vi "Dashboard Main.vi"() -> ()   [LabVIEW 2014]
uses:
  <vilib>/event_ctls.llb/eventvkey.ctl
  <vilib>/Rock Robotics/WPI/Dashboard/WPI_DashboardLogging Global.vi
  <vilib>/Rock Robotics/Network Tables/SD Read Number.vi
  <vilib>/Rock Robotics/Network Tables/SD Read Boolean Array.vi
  <vilib>/Rock Robotics/Network Tables/SD Read Boolean.vi
  <vilib>/Rock Robotics/Network Tables/SD Write Number.vi
  <vilib>/Rock Robotics/Network Tables/SD Write Boolean.vi
  <vilib>/Utility/config.llb/Write Key (String).vi
  <vilib>/Utility/config.llb/Write Key (I32).vi
  <vilib>/Utility/config.llb/NI_LVConfig.lvlib
panel:
  out "Gripper Open":bool
  out "Compresser Running":bool
  out "Camera 1":bool
  in  "TCP":refnum<k5>
  in  "Rec Mode":enum32{"Stop", "Record", "Playback"}(radio)
  in  "Vision":u16(ring)=2 items=["Camera Off", "USB Camera SW", "USB Camera HW", "IP Camera"]
  out "Camera IP":string
  out "Image Message":string="Timeout in Camera Communications"
  in  "Dashboard Tab":T1(tab)=enum."Drive"
  out "Inrange 2":bool
  out "Inrange 1":bool
  in  "Winch 2 Encoder reset":bool
  out "Lower Micro SW 2":bool
  out "Upper Micro SW 2":bool
  out "Manual Over-Rided Winch 2":bool=TRUE
  out "lower limit 2":dbl
  out "upper limit 2":dbl
  out "PV: 2":dbl(slide) scale=0.0..100.0
  in  "Winch 1 Encoder reset":bool
  out "Lower Micro SW":bool
  out "Upper Micro SW":bool
  out "Manual Over-Rided Winch 1":bool
  out "lower limit":dbl
  out "upper limit":dbl
  out "PV:":dbl(slide) scale=0.0..70.0
  out "SP:":dbl(slide) min=0.0 max=0.0 scale=0.0..75.0
  in  "Match Time":dbl=135.0
  out "Match Count Down":dbl=135.0 format="%#_4g"
  out "PICK UP":bool=TRUE
  out "Distance to Target":dbl(slide) scale=0.0..100.0
  in  "Autonomous Mode to run :":T2(ring)
  in  "Camera Settings":T3={"Frame Rate"=25, "Compression"=20, "Size"=0} {"Frame Rate" scale=1.0..30.0; "Size" items=["640x480", "320x240", "160x120"]}
  out "MotorChart R":cluster{"Numeric":dbl, "Numeric":dbl}(graph)
  out "MotorChart L":T4(graph)={"Numeric"=0.0, "Numeric"=0.0, "Battery V"=11.890625}
  out "MotorSliders R":cluster{"MotorSlide1":dbl, "MotorSlide2":dbl} {"MotorSlide2" scale=-1.0..1.0 scale format="%#_2e"; "MotorSlide1" scale=-1.0..1.0 scale format="%#_2e"}
  out "MotorSliders L":T5={"MotorSlide1"=0.0, "MotorSlide2"=0.0, "MotorSlide4 2"=11.890625} {"MotorSlide4 2" scale=0.0..14.0 scale format="%#_2e"; "MotorSlide2" scale=-1.0..1.0 scale format="%#_2e"; "MotorSlide1" scale=-1.0..1.0 scale format="%#_2e"}
  out "JS1 Z":dbl(slide) scale=-1.0..1.0 scale format="%#_2e"
  out "JS1 Graph":cluster{"X":dbl, "Y":dbl}[](graph)=[{"X"=0.047244094488188976, "Y"=-0.007874015748031496}]
  out "JS1 Buttons":T6
  out "JS2 Z":dbl(slide) scale=-1.0..1.0 scale format="%#_2e"
  out "JS2 Graph":cluster{"X":dbl, "Y":dbl}[](graph)=[{"X"=-0.015748031496062992, "Y"=-0.05511811023622047}]
  out "JS2 Buttons":T6
  out "Mode":T7(ring)
  in  "DB Camera Config":bool
  out "fps":dbl=13.440860215053762 format="%#.1g"
  out "Mbps":dbl=5.913673836823652 format="%#.1g"
  out "Mbps 2":bool
  out "Sonar Limit":dbl
  in  "DB/String 9":string
  in  "DB/String 8":string
  in  "DB/String 7":string
  in  "DB/String 6":string
  in  "DB/String 5":string
  in  "DB/String 4":string
  in  "DB/String 3":string
  in  "DB/String 2":string
  in  "DB/String 1":string
  in  "DB/String 0":string
  in  "DB/Slider 0":dbl(slide) scale=0.0..5.0
  in  "DB/Slider 1":dbl(slide) scale=0.0..5.0
  in  "DB/Slider 2":dbl(slide) scale=0.0..5.0
  in  "DB/Slider 3":dbl(slide) scale=0.0..5.0
  out "DB/LED 3":bool
  out "DB/LED 2":bool
  out "DB/LED 1":bool
  out "DB/LED 0":bool
  in  "DB/Button 3":bool
  in  "DB/Button 2":bool
  in  "DB/Button 1":bool
  in  "DB/Button 0":bool caption="New Name"
  in  "Test Slider":dbl(slide) scale=0.0..100.0 scale format="%#_3g"
  in  "On/Off":bool caption="Solenoid"
  in  "Test Name":u16(ring) items=["Select the test to run...", "Example Test", "-------------------------------", "List of tests is built in robot code.", "Replace with your own automated tests."]
  in  "Test Tree":string(tree)
  in  "Motor":cluster{"Value":dbl, "Enable":bool} {"Value" scale=-1.0..1.0 scale format="%#_3g"}
  out "Progress":T8 {"Test Progress" scale=0.0..100.0}
  in  "Rev/Fwd":cluster{"Forward":bool, "Reverse":bool}
  in  "Test Ring":u16(ring) items=["Monochrome", "Color"]
  in  "Listbox":i32(listbox)
  out "Tree":string(tree)
  out "Camera Image":T9(plugin-control)
  out "Boolean":bool=TRUE
  # "Left"
  # "Front"
  # "Right"
  # "Battery"
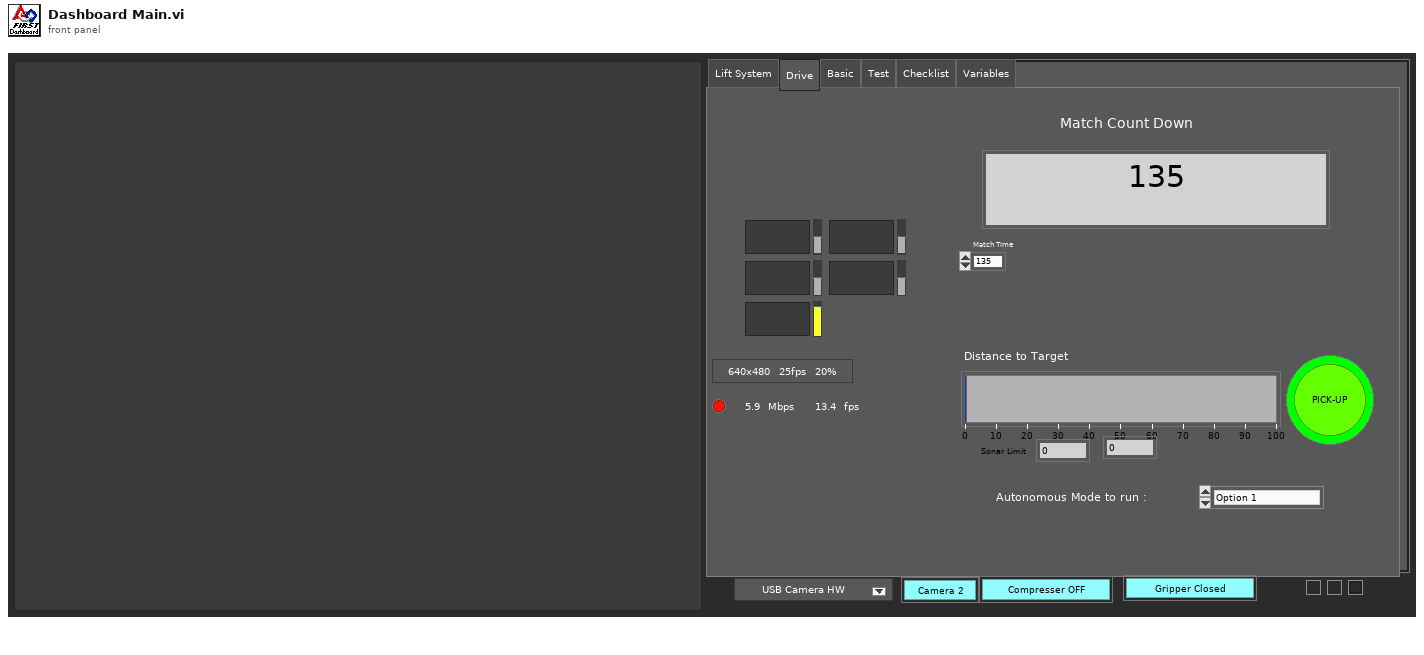
[diagram p1: front panel]
types:
  T1 = enum32{"Lift System", "Drive", "Basic", "Test", "Checklist", "Variables"}
  T2 = enum16{"Option 1", "Option 2", "Option 3", "Option 4", "Option 5", "Option 6"}
  T3 = cluster{"Frame Rate":i32, "Compression":i32, "Size":u16}
  T4 = cluster{"Numeric":dbl, "Numeric":dbl, "Battery V":dbl}
  T5 = cluster{"MotorSlide1":dbl, "MotorSlide2":dbl, "MotorSlide4 2":dbl}
  T6 = cluster{bool, bool, bool, bool, bool, bool, bool, bool, bool, bool, bool, bool}
  T7 = enum8{"Tele-Op Disabled", "Tele-Op Enabled", "Auto Disabled", "Auto Enabled", "Test Disabled", "Test Enabled", "Disconnected", "No Code", "E-Stop"}
  T8 = cluster{"Test Progress":u8, "Test Progress Text":string}
  T9 = typedef "IMAQ Image.ctl" = refnum<image>
  T10 = enum32{"Drive", "Basic", "Custom", "Test", "Checklist", "Variables"}
  T11 = typedef "Image Type" = u32
  T12 = cluster{"Camera Image":refnum<vi>, "Dashboard Tab":refnum<vi>, "Boolean":refnum<vi>, "Vision":refnum<vi>, "Rec Mode":refnum<vi>, "Test Slider":refnum<vi>, "On/Off ":refnum<vi>, "Test Ring":refnum<vi>, "Rev/Fwd":refnum<vi>, "Test Name":refnum<vi>, "Motor":refnum<vi>, "Progress":refnum<vi>, "CheckList":refnum<vi>, "Tree":refnum<vi>, "Test Tree":refnum<vi>}
  T13 = cluster{"Error Strings":string, "Disable Counts":cluster{u16, u16}, "Rail Faults":cluster{u16, u16, u16}, "Robot IP":string, "DB Mode":u8, "Event Info":cluster{"Name":string, "Type":u8, "Number":u16, "Replay":u8}, "Camera Addr":string}
  T14 = cluster{"Storage":cluster{"Disk Free":u64, "RAM Block":u32, "RAM free":u32}, "CPU Utilization":cluster{"CPU % ISR":sgl, "CPU % Time Crit":sgl, "CPU % Timed Str":sgl, "CPU % High":sgl, "CPU % Above":sgl, "CPU % Normal":sgl, "CPU % Low":sgl}, "CAN":cluster{"% Bus Utilization":sgl, "Bus Off Cnt":u32, "TX_FIFO Full Cnt":u32, "Receive Error Cnt":u8, "Transmit Error Cnt":u8}, "HID":cluster{"HID Outputs":u32, "Rumble Low":u16, "Rumble High":u16}[]}
  T15 = cluster{"Status bits":cluster{"Test Mode":bool, "Autonomous":bool, "Enabled":bool, "Code Start":bool, "Brownout":bool, "Reserved 2":bool, "Reserved 3":bool, "E-Stop":bool}, "Code Trace":cluster{"Disabled":bool, "TeleOp":bool, "Auto":bool, "Test":bool}, "Controller Type":enum16{"unknown", "cRIO", "roboRio"}, "Code?":enum16{"unknown", "noCode", "code"}, "Battery V":dbl}
  T16 = cluster{"Control Bits":cluster{"TestMode":bool, "Autonomous":bool, "Enabled":bool, "FMS Present":bool, bool, bool, bool, "E-Stop":bool}, "Team Station ":u8, "Countdown":sgl, "Joystick Values":cluster{"Axes":dbl[], "Buttons":bool[], "POVs":i16[]}[]}
  T17 = cluster{"Axes":dbl[], "Buttons":bool[], "POVs":i16[]}[]
  T18 = cluster{"Axes":dbl[], "Buttons":bool[], "POVs":i16[]}
  T19 = cluster{"Buttons[0]":bool, "Buttons[1]":bool, "Buttons[2]":bool, "Buttons[3]":bool, "Buttons[4]":bool, "Buttons[5]":bool, "Buttons[6]":bool, "Buttons[7]":bool, "Buttons[8]":bool, "Buttons[9]":bool, "Buttons[10]":bool, "Buttons[11]":bool}
  T20 = typedef "NI_LVConfig.lvlib/Config Data RefNum.ctl" = refnum<k1>
  T21 = cluster{"Operation":enum16{"Update", "Clear"}, "Color Box":u32}[]
  T22 = typedef "eventvkey.ctl" = enum16{"ASCII", "Enter", "Return", "Shift", "Ctrl", "Alt", "Cmd", "Opt", "Caps", "NumLock", "Clear", "Break", "Up", "Down", "Left", "Right", "Insert", "Delete", "Home", "End", "PageUp", "PageDown", "Escape", "Help", "Pause", "ScrollLock", "F1", "F2", "F3", "F4", "F5", "F6", "F7", "F8", "F9", "F10", "F11", "F12", "F13", "F14", "F15", "F16", "F17", "F18", "F19", "F20", "F21", "F22", "F23", "F24", "Play", "VolumeUp", "VolumeDown", "Mute", "Two Byte Char"}
  T23 = cluster{"Image Size":bool, "Image Type":bool, "Pixel Value":bool, "ROI Information":bool, "Zoom Factor":bool}
  T24 = enum8{"Enabled", "Disabled", "Disabled and Grayed Out"}
  T25 = cluster{"Operation":enum16{"Update", "Clear"}, "Color Box":u32}
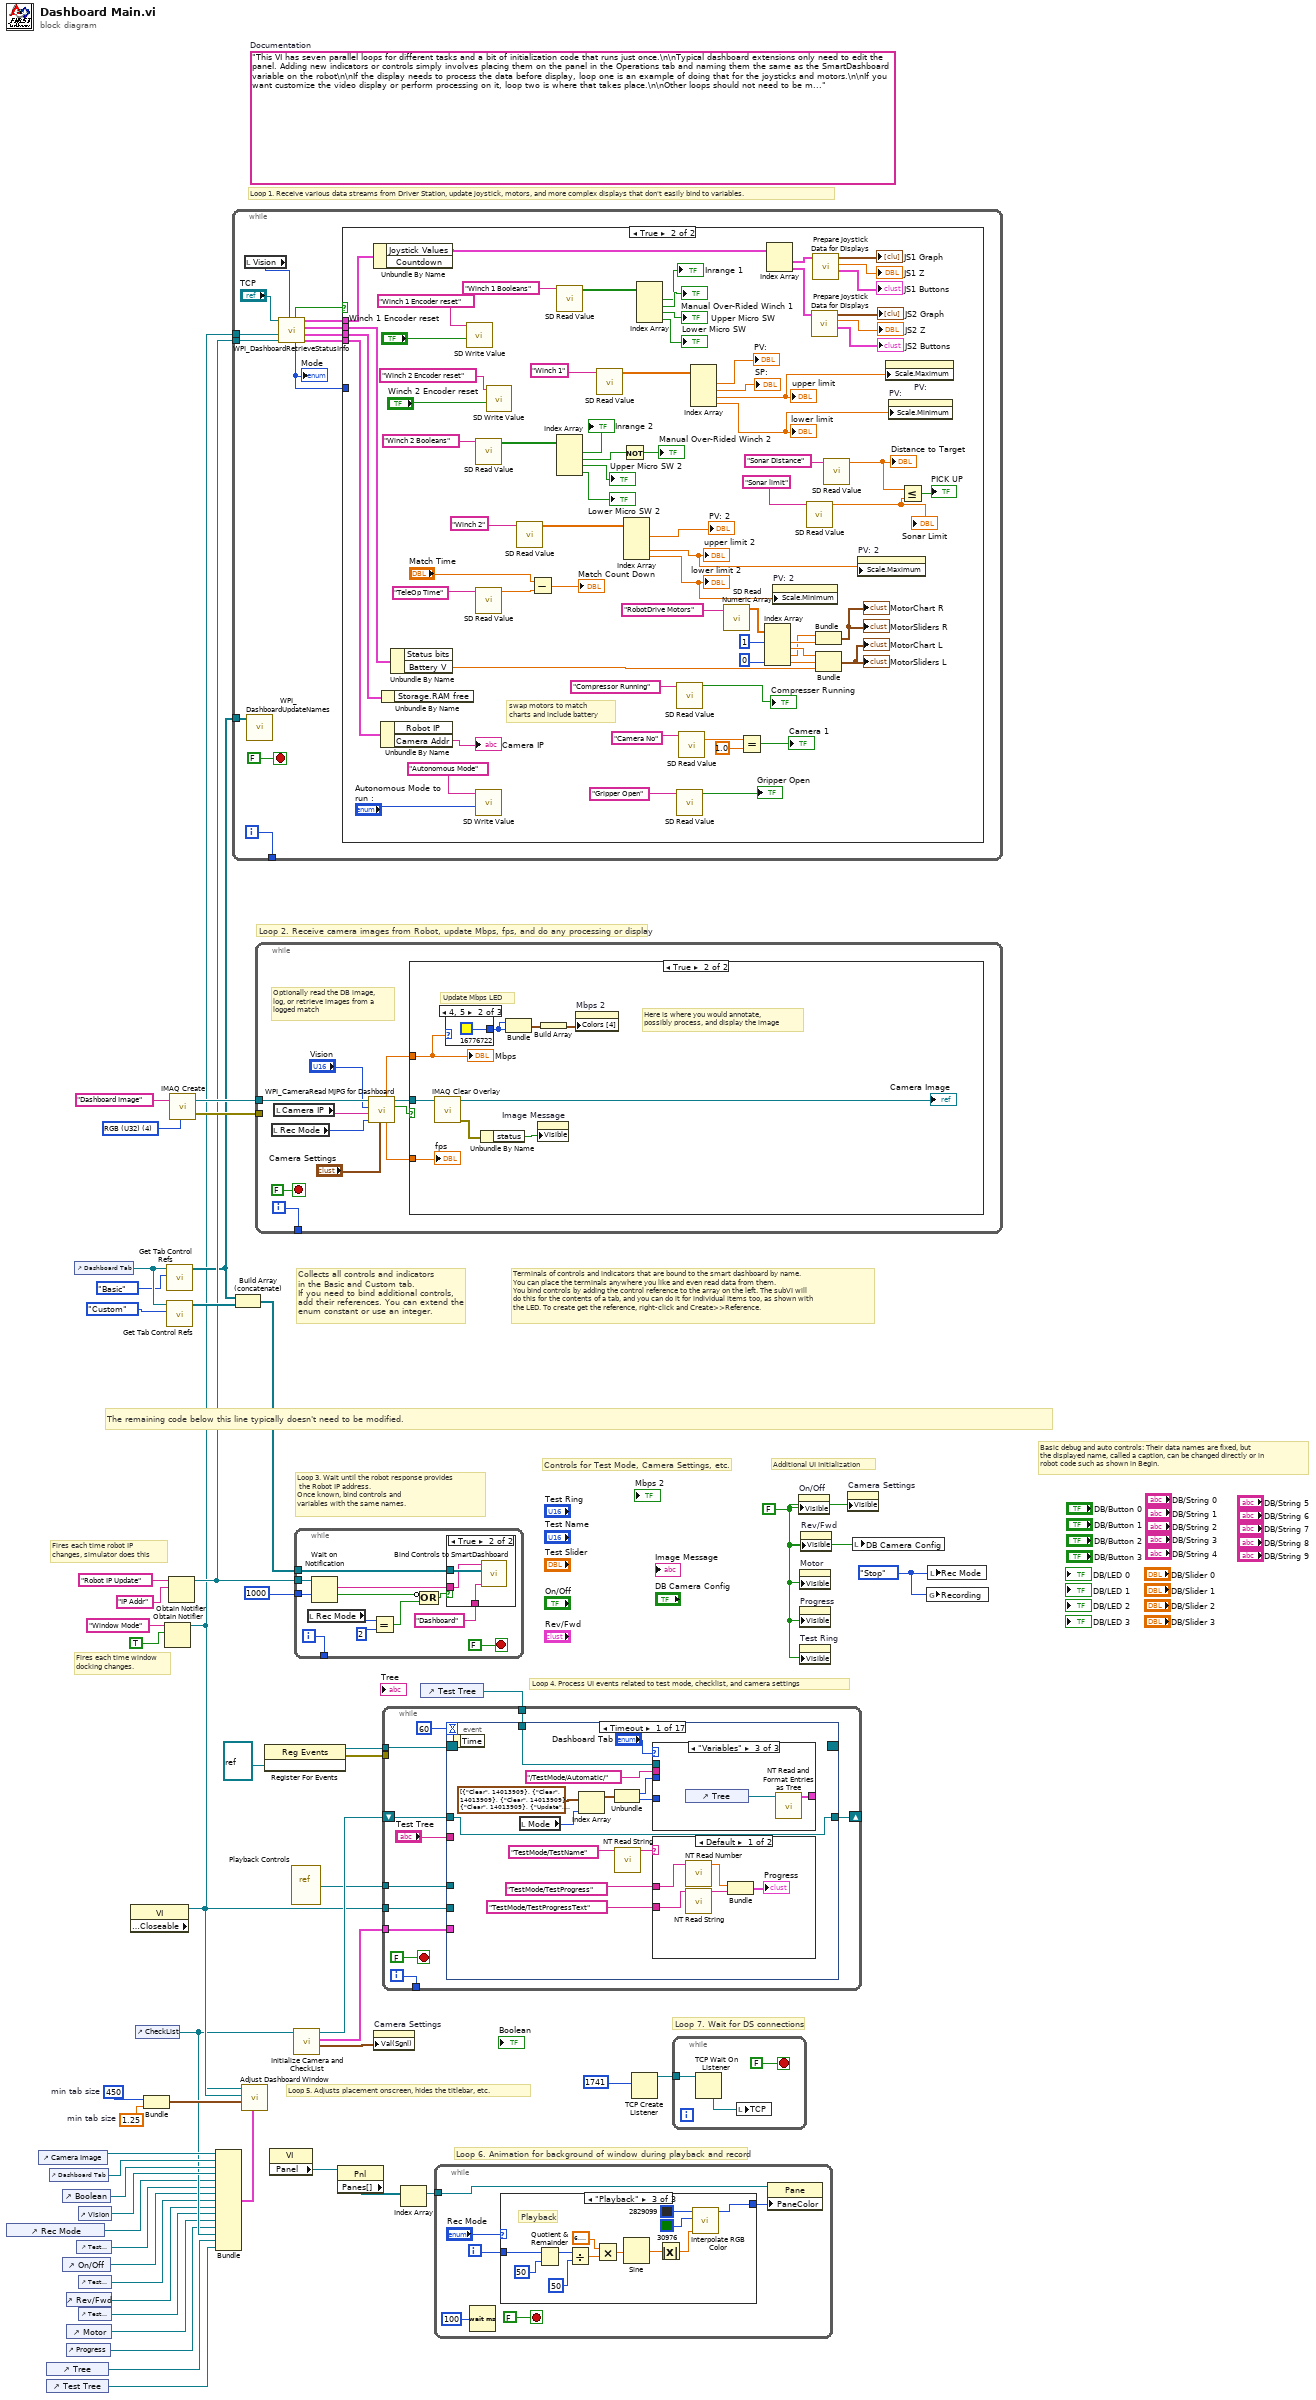
[diagram p0: block diagram]
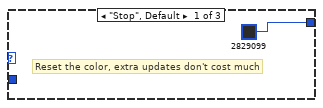
[diagram p3: hidden frame]
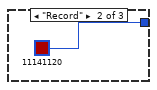
[diagram p4: hidden frame]
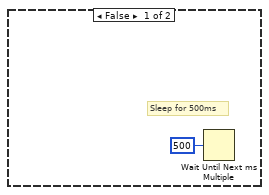
[diagram p6: hidden frame]
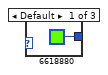
[diagram p7: hidden frame]
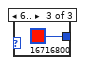
[diagram p8: hidden frame]
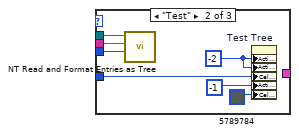
[diagram p10: hidden frame]
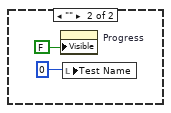
[diagram p11: hidden frame]
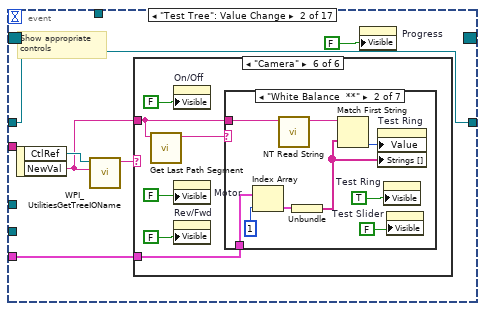
[diagram p12: hidden frame]
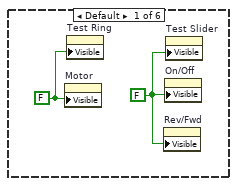
[diagram p13: hidden frame]
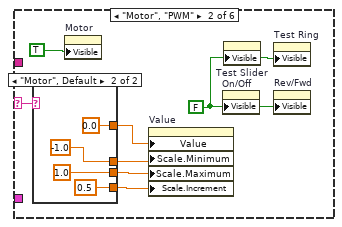
[diagram p14: hidden frame]
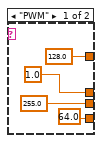
[diagram p15: hidden frame]
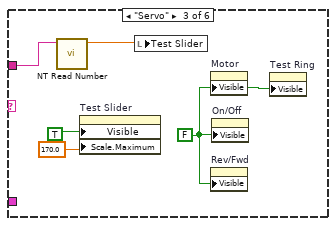
[diagram p16: hidden frame]
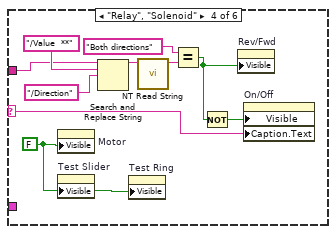
[diagram p17: hidden frame]
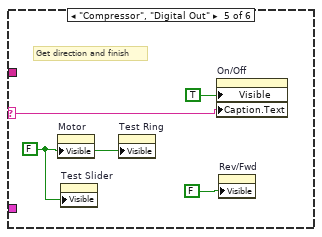
[diagram p18: hidden frame]
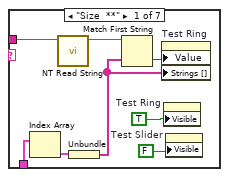
[diagram p19: hidden frame]
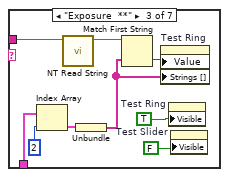
[diagram p20: hidden frame]
diagram:
  w24 = 450  # min tab size
  w23 = 1.25  # min tab size
  w32 = enum32{"Stop", "Record", "Playback"}."Stop" ("Rec Mode")
  w6 = FALSE ("Visible")
  (unwired) "This VI has seven parallel loops for different tasks and a bit of initialization code that runs just once.\n\nTypical dashboard extensions only need to edit the panel. Adding new indicators or controls simply involves placing them on the panel in the Operations tab and naming them the same as the SmartDashboard variable on the robot\n\nIf the display needs to process the data before display, loop one is an example of doing that for the joysticks and motors.\n\nIf you want customize the video display or perform processing on it, loop two is where that takes place.\n\nOther loops should not need to be modified. They are pretty standard, and document the task they perform."  # Documentation
  w52 = T11 4 items=["Grayscale (U8)", "Grayscale (I16)", "Grayscale (SGL)", "Complex (CSG)", "RGB (U32)", "HSL (U32)", "RGB (U64)"] ("Image Type")
  # "Loop 7. Wait for DS connections"
  # "Basic debug and auto controls: Their data names are fixed, but\nthe displayed name, called a caption, can be changed directly or in\nrobot code such as shown in Begin."
  # "Controls for Test Mode, Camera Settings, etc."
  # "Additional UI Initialization"
  # "Loop 6. Animation for background of window during playback and record"
  # "Fires each time robot IP\nchanges, simulator does this"
  # "Fires each time window\ndocking changes."
  # "Collects all controls and indicators\nin the Basic and Custom tab.\nIf you need to bind additional controls,\nadd their references. You can extend the\nenum constant or use an integer."
  # "The remaining code below this line typically doesn't need to be modified."
  # "Loop 4. Process UI events related to test mode, checklist, and camera settings"
  # "Terminals of controls and indicators that are bound to the smart dashboard by name.\nYou can place the terminals anywhere you like and even read data from them.\nYou bind controls by adding the control reference to the array on the left. The subVI will\ndo this for the contents of a tab, and you can do it for individual items too, as shown with\nthe LED. To create get the reference, right-click and Create>>Reference."
  # "Loop 3. Wait until the robot response provides\n the Robot IP address.\nOnce known, bind controls and\nvariables with the same names."
  # "Loop 5. Adjusts placement onscreen, hides the titlebar, etc."
  # "Loop 1. Receive various data streams from Driver Station, update joystick, motors, and more complex displays that don't easily bind to variables."
  # "Loop 2. Receive camera images from Robot, update Mbps, fps, and do any processing or display"
  n1 = control-ref of="Rec Mode"() -> (w12:refnum<vi>)
  n2 = control-ref of="Camera Image"() -> (w27:refnum<vi>)
  n3 = control-ref of="Tree"() -> (w16:refnum<vi>)
  n4 = control-ref of="Test Tree"() -> (w15:refnum<vi>)
  n5 = control-ref of="Dashboard Tab"() -> (w26:refnum<vi>)
  n6 = control-ref of="Boolean"() -> (w21:refnum<vi>)
  n7 = control-ref of="On/Off"() -> (w10:refnum<vi>)
  n8 = control-ref of="Progress"() -> (w7:refnum<vi>)
  n9 = control-ref of="Rev/Fwd"() -> (w8:refnum<vi>)
  n10 = control-ref of="Motor"() -> (w13:refnum<vi>)
  n11 = control-ref of="Dashboard Tab"() -> (w30:refnum<vi>)
  n12 = control-ref of="Test Slider"() -> (w11:refnum<vi>)
  n13 = control-ref of="Vision"() -> (w25:refnum<vi>)
  n14 = control-ref of="Test Ring"() -> (w9:refnum<vi>)
  n15 = control-ref of="Test Name"() -> (w14:refnum<vi>)
  n16 = property class="VI" props=["Front Panel.Closeable"]() -> (reference out=w31:refnum<vi>)  [unwired: 2 in, 2 out]
  n17 = control-ref of="CheckList"() -> (w17:refnum<vi>)
  n18 = Bundle("min tab size"=w24, "min tab size"=w23) -> (w22:cluster{"min tab size":i32, "min tab size":dbl})  [unwired: 1 in]
  n19 = Obtain Notifier(name (unnamed)="Window Mode", notification data type=TRUE) -> (notifier out=w3:refnum<notifier>)  [unwired: 2 in, 2 out]
  n20 = call <vilib>:"Get Tab Control Refs.vi"("Page Index"=T10."Basic" ("Dashboard Tab"), "TabControl in"=w30) -> ("ControlsOnPage"=w4:refnum<vi>[])  [unwired: 9 in]
  n21 = call <vilib>:"Get Tab Control Refs.vi"("Page Index"=T10."Custom" ("Dashboard Tab"), "TabControl in"=w30) -> ("ControlsOnPage"=w29:refnum<vi>[])  [unwired: 9 in]
  n22 = Obtain Notifier(name (unnamed)="Robot IP Update", notification data type="IP Addr" ("name (unnamed)")) -> (notifier out=w5:refnum<notifier>)  [unwired: 2 in, 2 out]
  n23 = call "IMAQ Create"("Image Name"="Dashboard Image", "Image Type"=w52) -> ("New Image"=w50:T9, "error out"=w49:errorcluster)  [unwired: 2 in, 1 out]
  n24 = Bundle("Camera Image"=w27, "Dashboard Tab"=w26, "Boolean"=w21, "Vision"=w25, "Rec Mode"=w12, "Test Slider"=w11, "On/Off"=w10, "Test Ring"=w9, "Rev/Fwd"=w8, "Test Name"=w14, "Motor"=w13, "Progress"=w7, "CheckList"=w17, "Tree"=w16, "Test Tree"=w15) -> (w18:T12)  [unwired: 1 in]
  n25 = while {
    tunnel: [w64] -> _
    tunnel: w5 -> [w58]
    tunnel: w4 -> [w57]
    tunnel: w3 -> [w53]
    i -> [w64]
    stop <- FALSE stop-if-true
    n26 = local read "Vision"() -> (w55:u16)
    n27 = call <vilib>:"WPI_DashboardUpdateNames.vi"("Controls on Tab"=w57) -> ()  [unwired: 11 in]
    n28 = call <vilib>:"WPI_DashboardRetrieveStatusInfo.vi"("Vision"=w55, "Binding Refnum"=w58, "Window Mode Notifier"=w53, "TCP Cnx"="TCP") -> ("Power and Errors"=w59:T13, "Robot Metrics"=w62:T14, "Status Info"=w63:T15, "Control Info"=w60:T16, "Robot Mode"=w56:T7, "Process?"=w61:bool)  [unwired: 2 in]
    "Mode" <- w56
    n29 = case shown="True" w61 {
      tunnel: w63 -> [_ w137]
      tunnel: w62 -> [_ w136]
      tunnel: w60 -> [_ w135]
      tunnel: w59 -> [_ w134]
      tunnel: w56 -> [_ _]
      frame False {
      }
      frame True {
        # "swap motors to match\ncharts and include battery"
        n30 = Unbundle By Name(w135) -> ("Joystick Values"=w122:T17)  [unwired: 1 out]
        n31 = Unbundle By Name(w134) -> ("Camera Addr"=→"Camera IP":string)  [unwired: 1 out]
        n32 = Unbundle By Name(w136) -> ()  [unwired: 1 out]
        n33 = Unbundle By Name(w137) -> ("Battery V"=w123:dbl)  [unwired: 1 out]
        n34 = call-poly <vilib>:"SD Write Value.vi"("Boolean"="Winch 1 Encoder reset", "Name"="Winch 1 Encoder reset") -> ()  [unwired: 8 in, 2 out]
        n35 = call-poly <vilib>:"SD Read Value.vi"("Name"="Winch 2 Booleans") -> ("Boolean Array"=w103:bool[])  [unwired: 8 in, 2 out]
        n36 = call-poly <vilib>:"SD Read Value.vi"("Name"="TeleOp Time") -> ("Numeric"=w70:dbl)  [unwired: 8 in, 2 out]
        n37 = call-poly <vilib>:"SD Write Value.vi"("Numeric"="Autonomous Mode to run :", "Name"="Autonomous Mode") -> ()  [unwired: 8 in, 2 out]
        n38 = call-poly <vilib>:"SD Write Value.vi"("Boolean"="Winch 2 Encoder reset", "Name"="Winch 2 Encoder reset") -> ()  [unwired: 8 in, 2 out]
        n39 = call-poly <vilib>:"SD Read Value.vi"("Name"="Winch 2") -> ("Numeric Array"=w101:dbl[])  [unwired: 8 in, 2 out]
        n40 = Subtract(x="Match Time", y=w70) -> (x-y=→"Match Count Down":dbl)
        n41 = call-poly <vilib>:"SD Read Value.vi"("Name"="Winch 1 Booleans") -> ("Boolean Array"=w106:bool[])  [unwired: 8 in, 2 out]
        n42 = Index Array(array=w103) -> (element #1=→"Inrange 2":bool, element #2=w97:bool, element #3=→"Upper Micro SW 2":bool, element #4=→"Lower Micro SW 2":bool)  [unwired: 4 in]
        n43 = call-poly <vilib>:"SD Read Value.vi"("Name"="Winch 1") -> ("Numeric Array"=w108:dbl[])  [unwired: 8 in, 2 out]
        n44 = Not(x=w97) -> (.not. x?=→"Manual Over-Rided Winch 2":bool)
        n45 = Index Array(array=w101) -> (element #1=→"PV: 2":dbl, element #3=w72:dbl, element #4=w71:dbl)  [unwired: 4 in, 1 out]
        "lower limit 2" <- w71
        "upper limit 2" <- w72
        n46 = Index Array(array=w106) -> (element #1=→"Inrange 1":bool, element #2=→"Manual Over-Rided Winch 1":bool, element #3=→"Upper Micro SW":bool, element #4=→"Lower Micro SW":bool)  [unwired: 4 in]
        n47 = call-poly <vilib>:"SD Read Value.vi"("Name"="Compressor Running") -> ("Boolean"=→"Compresser Running":bool)  [unwired: 8 in, 2 out]
        n48 = call-poly <vilib>:"SD Read Value.vi"("Name"="Gripper Open") -> ("Boolean"=→"Gripper Open":bool)  [unwired: 8 in, 2 out]
        n49 = call-poly <vilib>:"SD Read Value.vi"("Name"="Camera No") -> ("Numeric"=w109:dbl)  [unwired: 8 in, 2 out]
        n50 = Index Array(array=w108) -> (element #1=→"PV:":dbl, element #2=→"SP:":dbl, element #3=w74:dbl, element #4=w73:dbl)  [unwired: 4 in]
        "upper limit" <- w74
        "lower limit" <- w73
        n51 = call <vilib>:"SD Read Numeric Array.vi"("Name"="RobotDrive Motors") -> ("Numeric Array"=w125:dbl[])  [unwired: 8 in, 2 out]
        n52 = Equal?(x=w109, y=1.0) -> (x = y?=→"Camera 1":bool)
        n53 = Index Array(array=w125, index #1=1, index #4=0) -> (element #1=w129:dbl, element #2=w130:dbl, element #3=w128:dbl, element #4=w133:dbl)  [unwired: 2 in]
        n54 = Index Array(array=w122) -> (element #1=w121:T18, element #2=w116:T18)  [unwired: 2 in]
        n55 = property on="PV: 2" class="Slide (strict)"("Scale.Minimum"=w71) -> ()  [unwired: 2 in, 2 out]
        n56 = call-poly <vilib>:"SD Read Value.vi"("Name"="Sonar limit") -> ("Numeric"=w67:dbl)  [unwired: 8 in, 2 out]
        "Sonar Limit" <- w67
        n57 = call "Prepare Joystick Data for Displays.vi"("Joystick Values"=w116) -> ("Buttons"=→"JS2 Buttons":T19, "Z Axis"=→"JS2 Z":dbl, "Cartesian Data"=→"JS2 Graph":cluster{"X axis":dbl, "X axis":dbl}[])  [unwired: 8 in]
        n58 = call "Prepare Joystick Data for Displays.vi"("Joystick Values"=w121) -> ("Buttons"=→"JS1 Buttons":T19, "Z Axis"=→"JS1 Z":dbl, "Cartesian Data"=→"JS1 Graph":cluster{"X axis":dbl, "X axis":dbl}[])  [unwired: 8 in]
        n59 = Bundle("Numeric"=w128, "Numeric"=w129) -> (→"MotorChart R" →"MotorSliders R":cluster{"Numeric":dbl, "Numeric":dbl})  [unwired: 1 in]
        n60 = Bundle("Numeric"=w130, "Numeric"=w133, "Battery V"=w123) -> (→"MotorChart L" →"MotorSliders L":T4)  [unwired: 1 in]
        n61 = call-poly <vilib>:"SD Read Value.vi"("Name"="Sonar Distance") -> ("Numeric"=w84:dbl)  [unwired: 8 in, 2 out]
        "Distance to Target" <- w84
        n62 = property on="PV: 2" class="Slide (strict)"("Scale.Maximum"=w72) -> ()  [unwired: 2 in, 2 out]
        n63 = property on="PV:" class="Slide (strict)"("Scale.Maximum"=w74) -> ()  [unwired: 2 in, 2 out]
        n64 = property on="PV:" class="Slide (strict)"("Scale.Minimum"=w73) -> ()  [unwired: 2 in, 2 out]
        n65 = Less Or Equal?(x=w84, y=w67) -> (x <= y?=→"PICK UP":bool)
      }
    }
  }
  n66 = Build Array (concatenate)(w4, w29) -> (w28:refnum<vi>[])
  n67 = call "Adjust Dashboard Window.vi"("Sizing Refnums"=w18, "Size Constraints"=w22, "VI"=w31, "Notifier in"=w3) -> ()  [unwired: 8 in]
  n68 = while {
    tunnel: w50 -> [w146]
    tunnel: w49 -> [_]
    tunnel: [w147] -> _
    i -> [w147]
    stop <- FALSE stop-if-true
    # "Optionally read the DB image,\nlog, or retrieve images from a\nlogged match"
    n69 = local read "Rec Mode"() -> (w140:enum32{"Stop", "Record", "Playback"})
    n70 = local read "Camera IP"() -> (w138:string)
    n71 = call <vilib>:"WPI_CameraRead MJPG for Dashboard.vi"("Camera Settings"="Camera Settings", "Rec Mode"=w140, "Camera IP"=w138, "Camera Mode"="Vision", "Refnum in"=w146) -> ("Active"=w144:bool, "Refnum out"=w145:T9, "FPS"=w143:dbl, "Bandwidth (Mbps)"=w142:dbl)  [unwired: 3 in]
    n72 = case shown="True" w144 {
      tunnel: w145 -> [_ w153]
      tunnel: w142 -> [_ w152]
      tunnel: w143 -> [_ w150]
      frame False {
        # "Sleep for 500ms"
        n73 = Wait Until Next ms Multiple(millisecond multiple=u32 500) -> ()  [unwired: 1 out]
      }
      frame True {
        # "Here is where you would annotate,\npossibly process, and display the image"
        # "Update Mbps LED"
        n74 = call "IMAQ Clear Overlay"("Image"=w153) -> ("error out"=w157:errorcluster, "Image Out"=→"Camera Image":T9)  [unwired: 2 in, 7 out]
        n75 = case shown="4, 5" w152 {
          tunnel: [u32 6618880 ("Color Box") u32 16776722 ("Color Box") u32 16716800 ("Color Box")] -> w154
          frame Default {
          }
          frame 4, 5 {
          }
          frame 6.. {
          }
        }
        n76 = Unbundle By Name(w157) -> ("status"=w158:bool)
        n77 = Bundle("Color Box"=w154, "Color Box"=w154) -> (w156:cluster{"Color Box":u32, "Color Box":u32})  [unwired: 1 out]
        n78 = property on="Image Message" class="Str"("Visible"=w158) -> ()  [unwired: 2 in, 2 out]
        n79 = Build Array(w156) -> (w155:cluster{"Color Box":u32, "Color Box":u32}[])
        n80 = property on="Mbps 2" class="Bool (strict)"("Colors [4]"=w155) -> ()  [unwired: 2 in, 2 out]
        "Mbps" <- w152
        "fps" <- w150
      }
    }
  }
  n81 = register-events(refnum<vi> refnum) -> (reference out=w36:refnum<event-registration>, error out=w35:errorcluster)  [unwired: 2 in]
  n82 = property class="VI"() -> ("Panel"=w39:refnum<vi>)  [unwired: 2 in, 2 out]
  n83 = vi-ref "Playback Controls.vi"() -> (w37:refnum<vi>)
  n84 = call "Initialize Camera and CheckList.vi"("ListBox in"=w17) -> ("Cluster"=w43:cluster{"value":i32, "value":i32, "index":i32}, "Array"=w44:cluster{string[]}[], "File Refnum"=w42:T20)  [unwired: 8 in]
  n85 = while {
    tunnel: w28 -> [w173]
    tunnel: w5 -> [w171]
    tunnel: [w169] -> _
    tunnel: u32 1000 ("milliseconds to wait") -> [w168]
    i -> [w169]
    stop <- FALSE stop-if-true
    n86 = local read "Rec Mode"() -> (w164:enum32{"Stop", "Record", "Playback"})
    n87 = Wait on Notification(notifier=w171, timeout in ms (-1)=w168) -> (notification=w170:string, timed out?=w166:bool)  [unwired: 2 in, 2 out]
    n88 = Equal?(x=w164, y=u16 2 ("Rec Mode")) -> (x = y?=w165:bool)
    n89 = Compound Arithmetic op=OR(invert w166, w165) -> (w167:bool)
    n90 = case shown="True" w167 {
      tunnel: w173 -> [_ w176]
      tunnel: w170 -> [_ w175]
      tunnel: "Dashboard" -> [_ w174]
      frame False {
      }
      frame True {
        n91 = call <vilib>:"Bind Controls to SmartDashboard.vi"("Client Name"=w174, "Bound Control Refs"=w176, "Server IP Address"=w175) -> ()  [unwired: 9 in]
      }
    }
  }
  n92 = property class="Pnl"(reference=w39) -> ("Panes[]"=w40:refnum<vi>[])  [unwired: 1 in, 2 out]
  n93 = property on="Camera Settings" class="Clust (strict)"("Val(Sgnl)"=w43) -> ()  [unwired: 2 in, 2 out]
  n94 = Index Array(array=w40) -> (element=w38:refnum<vi>)  [unwired: 1 in]
  n95 = control-ref of="Test Tree"() -> (w41:refnum<vi>)
  n96 = while {
    tunnel: w44 -> [w184]
    shift-right: [w183] -> _
    shift-left: w42 -> [w182]
    tunnel: [w181] -> _
    tunnel: w41 -> [w180]
    tunnel: w37 -> [w179]
    tunnel: w36 -> [w178]
    tunnel: w35 -> [_]
    tunnel: w31 -> [w177]
    i -> [w181]
    stop <- FALSE stop-if-true
    n97 = event shown="[0] Timeout" {
      selector: w178 -> [_ _ _ _ _ _ _ _ _ _ _ _ _ _ _ _ _]
      dyn-events: [_ _ _ _ _ _ _ _ _ _ _ _ _ w422 _ _ _] -> _
      timeout: u32 60 ("milliseconds to wait") -> [_ _ _ _ _ _ _ _ _ _ _ _ _ _ _ _ _]
      tunnel: w180 -> [w197 _ _ _ _ _ _ _ _ _ _ _ _ _ _ _ _]
      tunnel: "Test Tree" -> [_ _ _ _ _ _ _ _ w391 w399 w401 w405 w413 _ _ _ _]
      tunnel: w184 -> [_ w218 _ _ _ _ w355 w385 _ _ _ _ _ _ _ _ _]
      tunnel: [w193 w217 w316 w321 w329 w341 w354 w378 w390 w397 w400 w404 w412 w424 w438 w439 w449] -> w183
      tunnel: w182 -> [w193 w217 w316 w321 w329 w341 w353 w378 w390 w397 w400 w404 w412 w424 w438 w439 w449]
      tunnel: w179 -> [_ _ _ _ _ _ _ _ _ _ _ _ _ w425 _ w442 _]
      tunnel: w177 -> [_ _ _ _ _ _ _ _ _ _ _ _ _ w420 _ _ _]
      event Timeout {
        n98 = event-data() -> ()  [unwired: 1 in, 1 out]
        n99 = local read "Mode"() -> (w196:T7)
        n100 = Index Array(array=T21 [{"Operation"=enum."Clear", "Color Box"=14013909}, {"Operation"=enum."Clear", "Color Box"=14013909}, {"Operation"=enum."Clear", "Color Box"=14013909}, {"Operation"=enum."Clear", "Color Box"=14013909}, {"Operation"=enum."Update", "Color Box"=14013909}, {"Operation"=enum."Update", "Color Box"=16777215}, {"Operation"=enum."Clear", "Color Box"=14013909}, {"Operation"=enum."Clear", "Color Box"=14013909}, {"Operation"=enum."Clear", "Color Box"=14013909}], index=w196) -> (element=w191:T25)
        n101 = Unbundle(w191) -> ("Operation"=w190:enum16{"Update", "Clear"}, "Color Box"=w189:u32)
        n102 = call <vilib>:"NT Read String.vi"("Name"="TestMode/TestName") -> ("String"=w199:string)  [unwired: 9 in, 1 out]
        n103 = case shown="\"Variables\"" "Dashboard Tab" {
          tunnel: w197 -> [_ w207 _]
          tunnel: "/TestMode/Automatic/" ("Name Pattern") -> [_ w206 _]
          tunnel: w190 -> [_ w205 _]
          tunnel: [_ _ w209] -> _
          tunnel: w189 -> [_ w201 _]
          frame "Lift System", Default {
          }
          frame "Test" {
            w204 = -2 ("Active Item:Row Number")
            n104 = call <vilib>:"NT Read and Format Entries as Tree.vi"("Operation"=w205, "Name Pattern"=w206, "Tree Refnum"=w207) -> ()  [unwired: 7 in, 2 out]
            n105 = property on="Test Tree" class="Tree (strict)"("Active Item Row Number"=w204, "ActiveColNum"=w204, "CellBG"=w201, "Active Item Row Number"=-1 ("Active Item:Row Number"), "CellBG"=u32 5789784 ("Color Box")) -> ()  [unwired: 2 in, 2 out]
          }
          frame "Variables" {
            n106 = control-ref of="Tree"() -> (w208:refnum<vi>)
            n107 = call <vilib>:"NT Read and Format Entries as Tree.vi"("Tree Refnum"=w208) -> ("Formatted Strings"=w209:cluster{"Name":string, "Value":string}[])  [unwired: 9 in, 1 out]
          }
        }
        n108 = case shown="Default" w199 {
          tunnel: "TestMode/TestProgress" ("Name") -> [w211 _]
          tunnel: "TestMode/TestProgressText" ("Name") -> [w210 _]
          frame Default {
            n109 = call <vilib>:"NT Read Number.vi"("Name"=w211) -> ("Numeric"=w212:dbl)  [unwired: 9 in, 1 out]
            n110 = call <vilib>:"NT Read String.vi"("Name"=w210) -> ("String"=w213:string)  [unwired: 9 in, 1 out]
            n111 = Bundle("Numeric"=w212, "String"=w213) -> (→"Progress":cluster{"Numeric":dbl, "String":string})  [unwired: 1 in]
          }
          frame "" {
            n112 = property on="Progress" class="Clust (strict)"("Visible"=FALSE) -> ()  [unwired: 2 in, 2 out]
            n113 = local write "Test Name"(u16 0) -> ()
          }
        }
      }
      event "Test Tree": Value Change {
        # "Show appropriate\ncontrols"
        n114 = event-data() -> ("CtlRef"=w221:refnum<vi>, "NewVal"=w219:string)  [unwired: 1 in]
        n115 = call <vilib>:"WPI_UtilitiesGetTreeIOName.vi"("NewVal"=w219, "TreeControl in"=w221) -> ("I/O Name"=w222:string)  [unwired: 9 in]
        n116 = case shown="\"Camera\"" w222 {
          selector: w222 -> [_ w229 _ w247 w256 _]
          tunnel: w219 -> [_ _ w244 w246 _ w263]
          tunnel: w218 -> [_ _ _ _ _ w262]
          frame Default {
            w224 = FALSE ("Visible")
            w223 = FALSE ("Visible")
            n117 = property on="Motor" class="Clust (strict)"("Visible"=w223) -> ()  [unwired: 2 in, 2 out]
            n118 = property on="Test Ring" class="Ring (strict)"("Visible"=w223) -> ()  [unwired: 2 in, 2 out]
            n119 = property on="Rev/Fwd" class="Clust (strict)"("Visible"=w224) -> ()  [unwired: 2 in, 2 out]
            n120 = property on="On/Off" class="Bool (strict)"("Visible"=w224) -> ()  [unwired: 2 in, 2 out]
            n121 = property on="Test Slider" class="Slide (strict)"("Visible"=w224) -> ()  [unwired: 2 in, 2 out]
          }
          frame "Motor", "PWM" {
            w230 = FALSE ("Visible")
            n122 = case shown="\"Motor\", Default" w229 {
              tunnel: [1.0 ("Value") -1.0 ("Value")] -> w228
              tunnel: [255.0 ("Value") 1.0 ("Value")] -> w227
              tunnel: [128.0 ("Value") 0.0 ("Value")] -> w226
              tunnel: [64.0 ("Value") 0.5 ("Value")] -> w225
              frame "PWM" {
              }
              frame "Motor", Default {
              }
            }
            n123 = property on="Motor" class="Clust (strict)"("Visible"=TRUE) -> ()  [unwired: 2 in, 2 out]
            n124 = property on="Value" class="Slide (strict)"("Value"=w226, "Scale.Minimum"=w228, "Scale.Maximum"=w227, "Scale.Increment"=w225) -> ()  [unwired: 2 in, 2 out]
            n125 = property on="On/Off" class="Bool (strict)"("Visible"=w230) -> ()  [unwired: 2 in, 2 out]
            n126 = property on="Test Slider" class="Slide (strict)"("Visible"=w230) -> ()  [unwired: 2 in, 2 out]
            n127 = property on="Test Ring" class="Ring (strict)"("Visible"=w230) -> ()  [unwired: 2 in, 2 out]
            n128 = property on="Rev/Fwd" class="Clust (strict)"("Visible"=w230) -> ()  [unwired: 2 in, 2 out]
          }
          frame "Servo" {
            w242 = FALSE ("Visible")
            n129 = call <vilib>:"NT Read Number.vi"("Name"=w244) -> ("Numeric"=w243:dbl)  [unwired: 9 in, 1 out]
            n130 = property on="Test Slider" class="Slide (strict)"("Visible"=TRUE, "Scale.Maximum"=170.0 ("Scale.Range:Maximum")) -> ()  [unwired: 2 in, 2 out]
            n131 = local write "Test Slider"(w243) -> ()
            n132 = property on="Motor" class="Clust (strict)"("Visible"=w242) -> ()  [unwired: 2 in, 2 out]
            n133 = property on="Rev/Fwd" class="Clust (strict)"("Visible"=w242) -> ()  [unwired: 2 in, 2 out]
            n134 = property on="On/Off" class="Bool (strict)"("Visible"=w242) -> ()  [unwired: 2 in, 2 out]
            n135 = property on="Test Ring" class="Ring (strict)"("Visible"=w242) -> ()  [unwired: 2 in, 2 out]
          }
          frame "Relay", "Solenoid" {
            w245 = FALSE ("Visible")
            n136 = property on="Motor" class="Clust (strict)"("Visible"=w245) -> ()  [unwired: 2 in, 2 out]
            n137 = property on="Test Slider" class="Slide (strict)"("Visible"=w245) -> ()  [unwired: 2 in, 2 out]
            n138 = Search and Replace String(input string=w246, search string="/Value  **", replace string="/Direction") -> (result string=w252:string)  [unwired: 5 in, 3 out]
            n139 = property on="Test Ring" class="Ring (strict)"("Visible"=w245) -> ()  [unwired: 2 in, 2 out]
            n140 = call <vilib>:"NT Read String.vi"("Name"=w252) -> ("String"=w250:string)  [unwired: 9 in, 1 out]
            n141 = Equal?(x="Both directions", y=w250) -> (x = y?=w248:bool)
            n142 = Not(x=w248) -> (.not. x?=w249:bool)
            n143 = property on="Rev/Fwd" class="Clust (strict)"("Visible"=w248) -> ()  [unwired: 2 in, 2 out]
            n144 = property on="On/Off" class="Bool (strict)"("Visible"=w249, "Caption.Text"=w247) -> ()  [unwired: 2 in, 2 out]
          }
          frame "Compressor", "Digital Out" {
            w255 = FALSE ("Visible")
            # "Get direction and finish"
            n145 = property on="Motor" class="Clust (strict)"("Visible"=w255) -> ()  [unwired: 2 in, 2 out]
            n146 = property on="Test Slider" class="Slide (strict)"("Visible"=w255) -> ()  [unwired: 2 in, 2 out]
            n147 = property on="Test Ring" class="Ring (strict)"("Visible"=w255) -> ()  [unwired: 2 in, 2 out]
            n148 = property on="On/Off" class="Bool (strict)"("Visible"=TRUE, "Caption.Text"=w256) -> ()  [unwired: 2 in, 2 out]
            n149 = property on="Rev/Fwd" class="Clust (strict)"("Visible"=FALSE) -> ()  [unwired: 2 in, 2 out]
          }
          frame "Camera" {
            n150 = call <vilib>:"Get Last Path Segment.vi"("String in"=w263) -> ("String out"=w264:string)  [unwired: 10 in]
            n151 = property on="On/Off" class="Bool (strict)"("Visible"=FALSE) -> ()  [unwired: 2 in, 2 out]
            n152 = property on="Motor" class="Clust (strict)"("Visible"=FALSE) -> ()  [unwired: 2 in, 2 out]
            n153 = property on="Rev/Fwd" class="Clust (strict)"("Visible"=FALSE) -> ()  [unwired: 2 in, 2 out]
            n154 = case shown="\"White Balance  **\"" w264 {
              tunnel: w263 -> [w270 w279 w288 w297 w306 _ w312]
              tunnel: w262 -> [w268 w276 w285 w294 w303 _ _]
              frame "Size  **" {
                n155 = Index Array(array=w268) -> (element=w267:cluster{string[]})  [unwired: 1 in]
                n156 = call <vilib>:"NT Read String.vi"("Name"=w270) -> ("String"=w269:string)  [unwired: 9 in, 1 out]
                n157 = Unbundle(w267) -> (w265:string[])
                n158 = Match First String(2:w265, 3:w269) -> (0:w266:i32)  [unwired: 1 out]
                n159 = property on="Test Ring" class="Ring (strict)"("Value"=w266, "Strings []"=w265) -> ()  [unwired: 2 in, 2 out]
                n160 = property on="Test Ring" class="Ring (strict)"("Visible"=TRUE) -> ()  [unwired: 2 in, 2 out]
                n161 = property on="Test Slider" class="Slide (strict)"("Visible"=FALSE) -> ()  [unwired: 2 in, 2 out]
              }
              frame "White Balance  **" {
                n162 = Index Array(array=w276, index=1) -> (element=w277:cluster{string[]})
                n163 = call <vilib>:"NT Read String.vi"("Name"=w279) -> ("String"=w278:string)  [unwired: 9 in, 1 out]
                n164 = Unbundle(w277) -> (w274:string[])
                n165 = Match First String(2:w274, 3:w278) -> (0:w273:i32)  [unwired: 1 out]
                n166 = property on="Test Ring" class="Ring (strict)"("Value"=w273, "Strings []"=w274) -> ()  [unwired: 2 in, 2 out]
                n167 = property on="Test Ring" class="Ring (strict)"("Visible"=TRUE) -> ()  [unwired: 2 in, 2 out]
                n168 = property on="Test Slider" class="Slide (strict)"("Visible"=FALSE) -> ()  [unwired: 2 in, 2 out]
              }
              frame "Exposure  **" {
                n169 = Index Array(array=w285, index=2) -> (element=w286:cluster{string[]})
                n170 = call <vilib>:"NT Read String.vi"("Name"=w288) -> ("String"=w287:string)  [unwired: 9 in, 1 out]
                n171 = Unbundle(w286) -> (w282:string[])
                n172 = Match First String(2:w282, 3:w287) -> (0:w283:i32)  [unwired: 1 out]
                n173 = property on="Test Ring" class="Ring (strict)"("Value"=w283, "Strings []"=w282) -> ()  [unwired: 2 in, 2 out]
                n174 = property on="Test Ring" class="Ring (strict)"("Visible"=TRUE) -> ()  [unwired: 2 in, 2 out]
                n175 = property on="Test Slider" class="Slide (strict)"("Visible"=FALSE) -> ()  [unwired: 2 in, 2 out]
              }
              frame "Exposure Priority  **" {
                n176 = Index Array(array=w294, index=3) -> (element=w295:cluster{string[]})
                n177 = call <vilib>:"NT Read String.vi"("Name"=w297) -> ("String"=w296:string)  [unwired: 9 in, 1 out]
                n178 = Unbundle(w295) -> (w291:string[])
                n179 = Match First String(2:w291, 3:w296) -> (0:w292:i32)  [unwired: 1 out]
                n180 = property on="Test Ring" class="Ring (strict)"("Value"=w292, "Strings []"=w291) -> ()  [unwired: 2 in, 2 out]
                n181 = property on="Test Ring" class="Ring (strict)"("Visible"=TRUE) -> ()  [unwired: 2 in, 2 out]
                n182 = property on="Test Slider" class="Slide (strict)"("Visible"=FALSE) -> ()  [unwired: 2 in, 2 out]
              }
              frame "Color Enable  **" {
                n183 = Index Array(array=w303, index=4) -> (element=w304:cluster{string[]})
                n184 = call <vilib>:"NT Read String.vi"("Name"=w306) -> ("String"=w305:string)  [unwired: 9 in, 1 out]
                n185 = Unbundle(w304) -> (w300:string[])
                n186 = Match First String(2:w300, 3:w305) -> (0:w301:i32)  [unwired: 1 out]
                n187 = property on="Test Ring" class="Ring (strict)"("Value"=w301, "Strings []"=w300) -> ()  [unwired: 2 in, 2 out]
                n188 = property on="Test Ring" class="Ring (strict)"("Visible"=TRUE) -> ()  [unwired: 2 in, 2 out]
                n189 = property on="Test Slider" class="Slide (strict)"("Visible"=FALSE) -> ()  [unwired: 2 in, 2 out]
              }
              frame Default {
                n190 = property on="Test Ring" class="Ring (strict)"("Visible"=FALSE) -> ()  [unwired: 2 in, 2 out]
                n191 = property on="Test Slider" class="Slide (strict)"("Visible"=FALSE) -> ()  [unwired: 2 in, 2 out]
              }
              frame "Brightness  **", "Color Level  **", "Compression  **", "FPS  **", "Sharpness  **" {
                n192 = call <vilib>:"NT Read Number.vi"("Name"=w312) -> ("Numeric"=w311:dbl)  [unwired: 9 in, 1 out]
                n193 = local write "Test Slider"(w311) -> ()
                n194 = property on="Test Ring" class="Ring (strict)"("Visible"=FALSE) -> ()  [unwired: 2 in, 2 out]
                n195 = property on="Test Slider" class="Slide (strict)"("Visible"=TRUE, "Scale.Maximum"=100.0 ("Scale.Range:Maximum")) -> ()  [unwired: 2 in, 2 out]
              }
            }
          }
        }
        n196 = property on="Progress" class="Clust (strict)"("Visible"=FALSE) -> ()  [unwired: 2 in, 2 out]
      }
      event "Test Name": Mouse Enter {
        # "Populate the ring with the list of tests"
        n197 = event-data() -> ()  [unwired: 1 in, 1 out]
        n198 = call <vilib>:"NT Read String Array.vi"("Name"="TestMode/TestList") -> ("String Array"=w320:string[])  [unwired: 9 in, 1 out]
        n199 = Build Array (concatenate)("Select the test to run...", w320) -> (w319:string[])
        n200 = property on="Test Name" class="Ring (strict)"("Strings []"=w319) -> ()  [unwired: 2 in, 2 out]
      }
      event "Test Name": Value Change {
        w322 = FALSE ("Visible")
        # "Tell the robot the test name to run"
        n201 = event-data() -> ("NewVal"=w326:u16)  [unwired: 1 in]
        n202 = property on="Test Name" class="Ring (strict)"() -> ("Strings []"=w327:string[])  [unwired: 2 in, 2 out]
        n203 = local write "Progress"(T8 {"Test Progress"=0, "Test Progress Text"=""} ("Progress")) -> ()
        n204 = Index Array(array=w327, index=w326) -> (element=w325:string)
        n205 = call <vilib>:"NT Write String.vi"("String"=w325, "Name"="TestMode/TestName") -> ()  [unwired: 9 in, 1 out]
        n206 = property on="Progress" class="Clust (strict)"("Visible"=TRUE) -> ()  [unwired: 2 in, 2 out]
        n207 = property on="Motor" class="Clust (strict)"("Visible"=w322) -> ()  [unwired: 2 in, 2 out]
        n208 = property on="Test Slider" class="Slide (strict)"("Visible"=w322) -> ()  [unwired: 2 in, 2 out]
        n209 = property on="On/Off" class="Bool (strict)"("Visible"=w322) -> ()  [unwired: 2 in, 2 out]
        n210 = property on="Rev/Fwd" class="Clust (strict)"("Visible"=w322) -> ()  [unwired: 2 in, 2 out]
        n211 = property on="Test Ring" class="Ring (strict)"("Visible"=w322) -> ()  [unwired: 2 in, 2 out]
      }
      event "Listbox": Double Click {
        # "Shift clears all"
        # "Update symbols on the listbox"
        n212 = event-data() -> ("PlatMods.Shift"=w330:bool, "Row"=w332:i32)  [unwired: 1 in]
        n213 = case shown="True" w330 {
          tunnel: w332 -> [w336 _]
          tunnel: 1 -> [w335 _]
          frame False {
            n214 = property on="Listbox" class="LstBox (strict)"() -> ("Item Symbols"=w334:i32[])  [unwired: 2 in, 2 out]
            n215 = Replace Array Subset(array=w334, new element=w335, index=w336) -> (w333:i32[])
            n216 = property on="Listbox" class="LstBox (strict)"("Item Symbols"=w333) -> ()  [unwired: 2 in, 2 out]
          }
          frame True {
            w337 = 0 ("Top Row")
            n217 = property on="Listbox" class="LstBox (strict)"() -> ("Number of Rows"=w339:u32)  [unwired: 2 in, 2 out]
            n218 = Initialize Array(0, w339) -> (w338:i32[])
            n219 = property on="Listbox" class="LstBox (strict)"("Top Row"=w337, "Value"=w337, "Item Symbols"=w338) -> ()  [unwired: 2 in, 2 out]
          }
        }
      }
      event "Listbox": Key Down {
        # "Update symbols on the listbox\nLeft and right keys check and uncheck"
        n220 = event-data() -> ("VKey"=w343:T22)  [unwired: 1 in]
        n221 = case shown="\"Left\", \"Right\"" w343 {
          selector: w343 -> [w348 _]
          tunnel: eventvkey."Left" ("VKey") -> [w346 _]
          frame "Left", "Right" {
            n222 = Equal?(x=w346, y=w348) -> (x = y?=w347:bool)
            n223 = Select(t=0, s=w347, f=1) -> (s? t:f=w349:i32)
            n224 = property on="Listbox" class="LstBox (strict)"() -> ("Item Symbols"=w352:i32[])  [unwired: 2 in, 2 out]
            n225 = Replace Array Subset(array=w352, new element=w349, index="Listbox") -> (w351:i32[])
            n226 = property on="Listbox" class="LstBox (strict)"("Item Symbols"=w351) -> ()  [unwired: 2 in, 2 out]
          }
          frame Default {
          }
        }
      }
      event "DB Camera Config": Value Change {
        # "Show or hide the cluster of controls, store in ini file"
        n227 = event-data() -> ("NewVal"=w356:bool)  [unwired: 1 in]
        n228 = case shown="False" w356 {
          tunnel: w355 -> [w365 _]
          tunnel: [w358 w376] -> w354
          tunnel: w353 -> [w357 w376]
          frame False {
            w372 = "Camera"
            w375 = FALSE ("Visible")
            n229 = local read "Camera Settings"() -> (w364:T3)
            n230 = Index Array(array=w365) -> (element=w368:cluster{string[]})  [unwired: 1 in]
            n231 = Unbundle(w364) -> ("Frame Rate"=w363:i32, "Compression"=w362:i32, "Size"=w366:u16)
            n232 = Unbundle(w368) -> (w367:string[])
            n233 = Index Array(array=w367, index=w366) -> (element=w361:string)
            n234 = call-poly <vilib>:"Write Key.vi"("section"=w372, "value"=w361, "key"="Size", "refnum"=w357) -> ("refnum out"=w374:T20)  [unwired: 2 in, 5 out]
            n235 = call-poly <vilib>:"Write Key.vi"("section"=w372, "value"=w363, "key"="FrameRate", "refnum"=w374) -> ("refnum out"=w373:T20)  [unwired: 1 in, 6 out]
            n236 = property on="Camera Settings" class="Clust (strict)"("Visible"=w375) -> ()  [unwired: 2 in, 2 out]
            n237 = local write "DB Camera Config"(w375) -> ()
            n238 = call-poly <vilib>:"Write Key.vi"("section"=w372, "value"=w362, "key"="Compression", "refnum"=w373) -> ("refnum out"=w359:T20)  [unwired: 1 in, 6 out]
            n239 = call <vilib>:"Close Config Data.vi"("refnum"=w359) -> ("file path"=w360:path)  [unwired: 2 in, 8 out]
            n240 = call <vilib>:"Open Config Data.vi"("configuration file path"=w360) -> ("refnum"=w358:T20)  [unwired: 8 in, 2 out]
          }
          frame True {
            n241 = property on="Camera Settings" class="Clust (strict)"("Visible"=TRUE) -> ()  [unwired: 2 in, 2 out]
          }
        }
      }
      event "Camera Settings": Value Change {
        # "Update summary string when any elements of DB camera change"
        n242 = event-data() -> ("NewVal"=w389:T3)  [unwired: 1 in]
        n243 = Index Array(array=w385) -> (element=w384:cluster{string[]})  [unwired: 1 in]
        n244 = Unbundle(w389) -> ("Frame Rate"=w380:i32, "Compression"=w379:i32, "Size"=w382:u16)
        n245 = Unbundle(w384) -> (w383:string[])
        n246 = Index Array(array=w383, index=w382) -> (element=w381:string)
        n247 = Format Into String(format string="%s   %dfps   %d%%", w381, w380, w379) -> (resulting string=w386:string)  [unwired: 2 in, 1 out]
        n248 = Build Array(w386) -> (w387:string[])
        n249 = property on="DB Camera Config" class="Bool (strict)"("Strings [4]"=w387) -> ()  [unwired: 2 in, 2 out]
      }
      event "Motor.Enable": Value Change {
        # "When the test mode otor enable helper is set, update that\ntree row item's value"
        n250 = event-data() -> ("NewVal"=w395:bool)  [unwired: 1 in]
        n251 = Unbundle("Motor") -> ("Value"=w394:dbl)  [unwired: 1 out]
        n252 = Select(t=w394, s=w395, f=0.0) -> (s? t:f=w392:dbl)
        n253 = call <vilib>:"NT Write Number.vi"("Numeric"=w392, "Name"=w391) -> ()  [unwired: 9 in, 1 out]
      }
      event "Test Slider": Value Change {
        # "When the test mode slider helper is set, update that\ntree row item's value"
        n254 = event-data() -> ("NewVal"=w398:dbl)  [unwired: 1 in]
        n255 = call <vilib>:"NT Write Number.vi"("Numeric"=w398, "Name"=w399) -> ()  [unwired: 9 in, 1 out]
      }
      event "On/Off": Value Change {
        # "When the test mode on/off helper value is set, update that\ntree row item's value"
        n256 = event-data() -> ("NewVal"=w403:bool)  [unwired: 1 in]
        n257 = Boolean To (0,1)(Boolean=w403) -> (0, 1=w402:i16)
        n258 = call <vilib>:"NT Write Number.vi"("Numeric"=w402, "Name"=w401) -> ()  [unwired: 9 in, 1 out]
      }
      event "Rev/Fwd": Value Change {
        # "When the test mode helper value for relays is set, update that\ntree row item's value"
        n259 = event-data() -> ("NewVal.Forward"=w411:bool, "NewVal.Reverse"=w410:bool)  [unwired: 1 in]
        n260 = Boolean To (0,1)(Boolean=w411) -> (0, 1=w407:i16)
        n261 = Boolean To (0,1)(Boolean=w410) -> (0, 1=w409:i16)
        n262 = Negate(x=w409) -> (-x=w408:i16)
        n263 = Add(x=w407, y=w408) -> (x+y=w406:i16)
        n264 = call <vilib>:"NT Write Number.vi"("Numeric"=w406, "Name"=w405) -> ()  [unwired: 9 in, 1 out]
      }
      event "Test Ring": Value Change {
        # "When a test mode helper value is selected from the ring,\nset the tree item's variable to the string value"
        n265 = event-data() -> ("NewVal"=w415:u16)  [unwired: 1 in]
        n266 = property on="Test Ring" class="Ring (strict)"() -> ("Strings []"=w416:string[])  [unwired: 2 in, 2 out]
        n267 = Index Array(array=w416, index=w415) -> (element=w414:string)
        n268 = call <vilib>:"NT Write String.vi"("String"=w414, "Name"=w413) -> ()  [unwired: 9 in, 1 out]
      }
      event "Rec Mode": Value Change {
        # "Update globals for recording mode and path to read log from.\nClear when logging and let NetworkTables set path for vision to\nuse."
        n269 = event-data() -> ("NewVal"=w426:enum32{"Stop", "Record", "Playback"})  [unwired: 1 in]
        n270 = case shown="\"Playback\"" w426 {
          tunnel: w425 -> [_ w428 w436]
          tunnel: [_ _ w435] -> w422
          tunnel: [_ _ w434] -> _
          tunnel: w420 -> [_ _ w432]
          tunnel: cluster{i32, i32} {-250, 170} -> [_ _ w431]
          tunnel: [_ _ T23 {"Image Size"=TRUE, "Image Type"=TRUE, "Pixel Value"=TRUE, "ROI Information"=TRUE, "Zoom Factor"=FALSE} ("Image Information Shown:All Elements")] -> w418
          tunnel: [_ _ TRUE ("Zoom Factor")] -> w417
          frame Default {
          }
          frame "Stop", "Record" {
            # "Place Window too"
            n271 = invoke class="VI" method="FP.Close"(reference=w428) -> (reference out=w427:refnum<vi>)  [unwired: 2 in, 2 out]
            n272 = invoke class="VI" method="Abort VI"(reference=w427) -> ()  [unwired: 2 in, 3 out]
          }
          frame "Playback" {
            n273 = call "Open Playback Panel.vi"("Offset"=w431, "DB VI Ref"=w432, "Playback in"=w436) -> ("Playback out"=w433:refnum<vi>)  [unwired: 8 in]
            n274 = register-events(w433) -> (reference out=w435:refnum<event-registration>, error out=w434:errorcluster)  [unwired: 2 in]
          }
        }
        n275 = global write "WPI_DashboardLogging Global.vi" "Recording"(w426) -> ()
        n276 = global write "WPI_DashboardLogging Global.vi" "Logging Filename"(path "") -> ()
        n277 = property on="Camera Image" class="ImageControl"("Image Information Shown"=w418, "Image Information Visible"=w417) -> ()  [unwired: 2 in, 2 out]
        n278 = call <vilib>:"WPI_DashboardNT Log FieldName Cache.vi"("Operation"=enum16{"Lookup/Add", "Index", "Clear"}."Clear") -> ()  [unwired: 8 in, 3 out]
      }
      event Panel Close {
        w437 = enum32{"Stop", "Record", "Playback"}."Stop" ("Rec Mode")
        # "Playback window has been closed, abort"
        n279 = event-data() -> ()  [unwired: 1 in, 4 out]
        n280 = local write "Rec Mode"(w437) -> ()
        n281 = global write "WPI_DashboardLogging Global.vi" "Recording"(w437) -> ()
      }
      event Panel Close {
        # "Abort playback window and ourself"
        n282 = event-data() -> ()  [unwired: 1 in, 4 out]
        n283 = invoke class="VI" method="FP.Close"(reference=w442) -> (reference out=w441:refnum<vi>)  [unwired: 2 in, 2 out]
        n284 = invoke class="VI" method="Abort VI"(reference=w441) -> (error out=w440:errorcluster)  [unwired: 2 in, 2 out]
        n285 = invoke class="VI" method="Abort VI"(error in=w440) -> ()  [unwired: 2 in, 3 out]
      }
      event "Vision": Value Change {
        # "Enable/Disable Compression slider.\nHW USB is hard-coded into the camera"
        n286 = event-data() -> ("NewVal"=w448:u16)  [unwired: 1 in]
        n287 = Equal?(x=w448, y=u32 2 ("milliseconds to wait")) -> (x = y?=w446:bool)
        n288 = Select(t=T24."Disabled and Grayed Out" ("Disabled"), s=w446, f=T24."Enabled" ("Disabled")) -> (s? t:f=w443:T24)
        n289 = property on="Compression" class="Slide (strict)"("DisabledEnum"=w443) -> ()  [unwired: 2 in, 2 out]
      }
    }
  }
  n290 = while {
    tunnel: w38 -> [w451]
    i -> [w454]
    stop <- FALSE stop-if-true
    n291 = Wait (ms)(milliseconds to wait=u32 100) -> ()  [unwired: 1 out]
    n292 = case shown="\"Playback\"" "Rec Mode" {
      tunnel: w454 -> [_ _ w469]
      tunnel: [u32 2829099 ("Base Color") u32 11141120 ("Target Color") w458] -> w450
      frame "Stop", Default {
        # "Reset the color, extra updates don't cost much"
      }
      frame "Record" {
      }
      frame "Playback" {
        # "Playback"
        n293 = Quotient & Remainder(x=w469, y=u32 50 ("milliseconds to wait")) -> (x-y*floor(x/y)=w465:u32)  [unwired: 1 out]
        n294 = Divide(x=w465, y=u32 50 ("milliseconds to wait")) -> (x/y=w462:dbl)
        n295 = Multiply(x=6.283185307179586, y=w462) -> (x*y=w467:dbl)
        n296 = Sine(x=w467) -> (sin(x)=w466:dbl)
        n297 = Absolute Value(x=w466) -> (abs(x)=w459:dbl)
        n298 = call "Interpolate RGB Color.vi"("Proportion"=w459, "Target Color"=u32 30976, "Base Color"=u32 2829099) -> ("Result Color"=w458:u32)  [unwired: 8 in]
      }
    }
    n299 = property class="Pane"(reference=w451, "PaneColor"=w450) -> ()  [unwired: 1 in, 2 out]
  }
  n300 = TCP Create Listener(10:u16 1741 ("timeout ms (25000)")) -> (3:w1:refnum<k5>)  [unwired: 4 in, 2 out]
  n301 = while {
    tunnel: w1 -> [w471]
    stop <- FALSE stop-if-true
    n302 = TCP Wait On Listener(11:w471) -> (4:w470:refnum<k5>)  [unwired: 3 in, 4 out]
    n303 = local write "TCP"(w470) -> ()
  }
  n304 = property on="On/Off" class="Bool (strict)"("Visible"=w6) -> ()  [unwired: 2 in, 2 out]
  n305 = property on="Motor" class="Clust (strict)"("Visible"=w6) -> ()  [unwired: 2 in, 2 out]
  n306 = property on="Progress" class="Clust (strict)"("Visible"=w6) -> ()  [unwired: 2 in, 2 out]
  n307 = property on="Test Ring" class="Ring (strict)"("Visible"=w6) -> ()  [unwired: 2 in, 2 out]
  n308 = property on="Rev/Fwd" class="Clust (strict)"("Visible"=w6) -> ()  [unwired: 2 in, 2 out]
  n309 = property on="Camera Settings" class="Clust (strict)"("Visible"=w6) -> ()  [unwired: 2 in, 2 out]
  n310 = local write "DB Camera Config"(w6) -> ()
  n311 = global write "WPI_DashboardLogging Global.vi" "Recording"(w32) -> ()
  n312 = local write "Rec Mode"(w32) -> ()
